vi "Project Tree Update Step Display.vi"(8 "error in (no error)":errorcluster, 10 "Step Info":cluster{"Id":string, "Name":string, "Skip":bool}, 11 "Editor.lvclass in":refnum<data-value>) -> (0 "error out":errorcluster, 3 "Editor.lvclass out":refnum<data-value>)   [LabVIEW 2015, in "Editor.lvclass"]
uses:
  Editor.lvclass
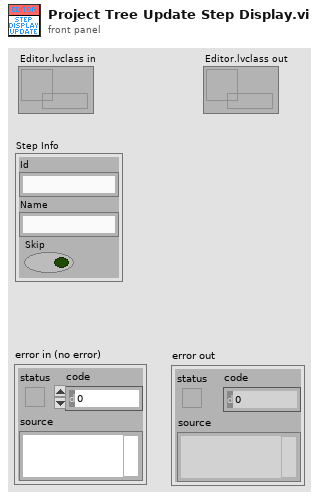
[diagram p1: front panel]
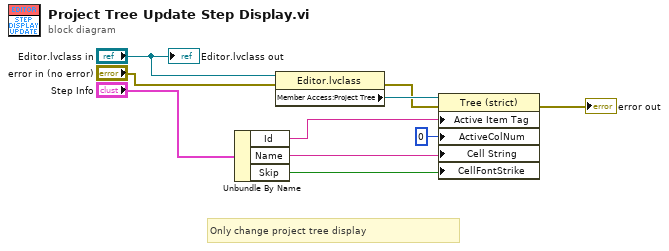
[diagram p0: block diagram]
diagram:
  # "Only change project tree display"
  n1 = Unbundle By Name("Step Info") -> ("Id"=w8:string, "Name"=w6:string, "Skip"=w5:bool)
  n2 = property class="Editor.lvclass"(reference="Editor.lvclass in", error in="error in (no error)") -> (error out=w3:errorcluster, "Member Access:Project Tree"=w10:refnum<vi>)  [unwired: 1 out]
  n3 = property class="Tree (strict)"(reference=w10, error in=w3, "Active Item Tag"=w8, "ActiveColNum"=0 ("Active Cell:Active Column Number"), "Cell String"=w6, "CellFontStrike"=w5) -> (error out=→"error out":errorcluster)  [unwired: 1 out]
  "Editor.lvclass out" <- "Editor.lvclass in"
